vi "Delayed Send.vi"(6 "Delay ms":i32, 7 "High Priority (F)":bool, 8 "error in (no error)":errorcluster, 9 "Data":variant, 10 "ID":string, 11 "MessageQ in":refnum<class "MessageQ.lvclass">) -> (0 "error out":errorcluster, 3 "MessageQ out":refnum<class "MessageQ.lvclass">)   [LabVIEW 2020, in "Volatus.lvlib" / "MessageQ.lvclass"]
uses:
  MessageQ.lvclass
  MessageQ.lvclass/MessageQ.ctl
  Delayed Send Async.vi
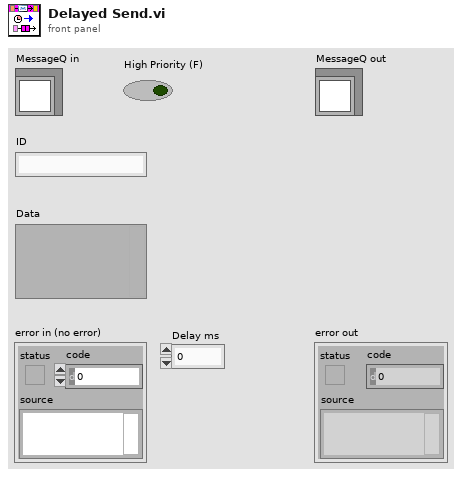
[diagram p1: front panel]
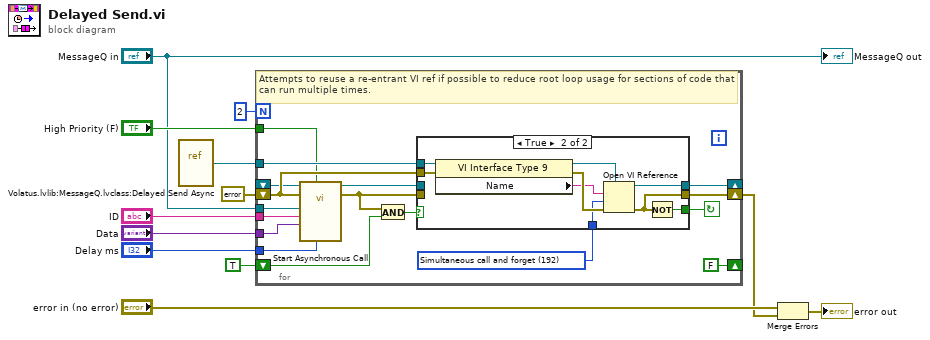
[diagram p0: block diagram]
diagram:
  n1 = vi-ref "Volatus.lvlib:MessageQ.lvclass:Delayed Send Async.vi"() -> (w9:refnum<vi>)
  n2 = for {
    N: 2 -> [_]
    tunnel: w9 -> [w28]
    shift-right: [w27] -> _
    shift-left: _ -> [w26]
    shift-right: [w24] -> w1
    shift-left: errorcluster {"status"=FALSE, "code"=0, "source"=""} ("error constant") -> [w29]
    shift-right: [FALSE] -> _
    shift-left: TRUE -> [w21]
    tunnel: "Delay ms" -> [w17]
    tunnel: "Data" -> [w16]
    tunnel: "ID" -> [w15]
    tunnel: "High Priority (F)" -> [w14]
    tunnel: "MessageQ in" -> [w13]
    stop <- w20 continue-if-true
    w18 = 192 items=["Record modifications"=1, "Open templates for editing"=2, "Prompt user to save"=4, "Prepare for reentrant run"=8, "Prompt to find missing subVIs"=16, "Hide loading dialog box"=32, "Enable simultaneous calls"=64, "Prepare to call and forget"=128, "Simultaneous call and forget"=192, "Prepare to call and collect"=256, "Simultaneous call and collect"=320]
    # "Attempts to reuse a re-entrant VI ref if possible to reduce root loop usage for sections of code that can run multiple times."
    n3 = call-by-ref "Start Asynchronous Call"(reference=w26, error in=w29, "Delay ms"=w17, "High Priority (F)"=w14, "Data"=w16, "ID"=w15, "MessageQ in"=w13) -> (reference out=w25:refnum<vi>, error out=w23:errorcluster)  [unwired: 7 in]
    n4 = And(x=w23, y=w21) -> (x .and. y?=w22:bool)
    n5 = case shown="True" w22 {
      tunnel: w28 -> [_ w39]
      tunnel: w18 -> [_ w37]
      tunnel: [w31 w35] -> w27
      tunnel: w25 -> [w31 _]
      tunnel: [w30 w33] -> w24
      tunnel: w23 -> [w30 _]
      tunnel: w29 -> [_ w34]
      tunnel: [_ w32] -> w20
      frame False {
      }
      frame True {
        n6 = property class="VI Interface Type 9"(reference=w39, error in=w34) -> (reference out=w36:refnum<vi>, error out=w40:errorcluster, "Name"=w38:string)
        n7 = Open VI Reference(type specifier VI Refnum (for type only)=w36, vi path=w38, options=w37, error in (no error)=w40) -> (vi reference=w35:refnum<vi>, error out=w33:errorcluster)  [unwired: 2 in]
        n8 = Not(x=w33) -> (.not. x?=w32:bool)
      }
    }
  }
  n9 = Merge Errors("error in (no error)", w1) -> (→"error out":errorcluster)
  "MessageQ out" <- "MessageQ in"
